vi "MeasurementServer_FourProbeMeasurement_WriteValue.vi"(0 "gRPCid":T3, 1 "FourProbeRawData":T1, 3 "error in (no error)":errorcluster) -> (10 "error out":errorcluster)   [LabVIEW 2019, in "labview-grpc-measurement-server.lvlib"]
uses:
  labview-grpc-measurement-server.lvlib
  MeasurementServer_gRPCid.ctl
  MeasurementServer_FourProbeRawData.ctl
  MeasurementServer_ErrorOutData.ctl
  <vilib>/Utility/error.llb/Error Cluster From Error Code.vi
  <vilib>/ErrorRing/Error Ring.xnode
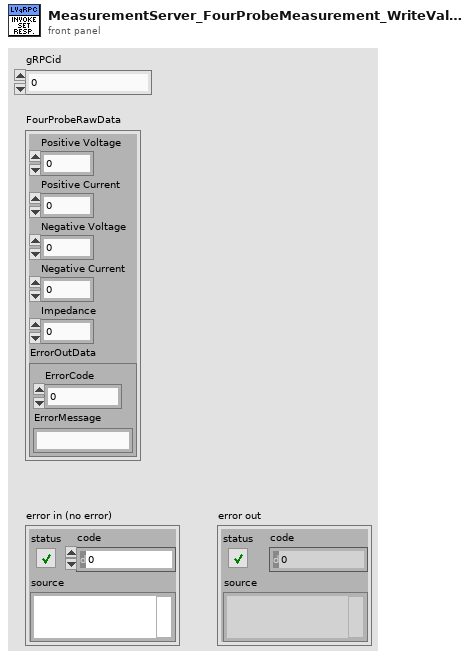
[diagram p1: front panel]
types:
  T1 = typedef "labview-grpc-measurement-server.lvlib/MeasurementServer_FourProbeRawData.ctl" = cluster{"Positive Voltage":dbl, "Positive Current":dbl, "Negative Voltage":dbl, "Negative Current":dbl, "Impedance":dbl, "ErrorOutData":T2}
  T2 = typedef "labview-grpc-measurement-server.lvlib/MeasurementServer_ErrorOutData.ctl" = cluster{"ErrorCode":i32, "ErrorMessage":string}
  T3 = typedef "labview-grpc-measurement-server.lvlib/MeasurementServer_gRPCid.ctl" = u64
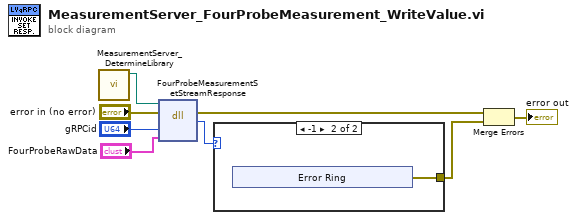
[diagram p0: block diagram]
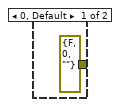
[diagram p2: hidden frame]
diagram:
  n1 = call "MeasurementServer_DetermineLibrary.vi"() -> ("path out"=w1:path)  [unwired: 11 in]
  n2 = dll-call lib="C:/dev/labview-grpc-measurement-server/build/Debug/labview_measurement_server.dll" fn="FourProbeMeasurementSetStreamResponse"(path in=w1, error in="error in (no error)", "id"="gRPCid", "data"="FourProbeRawData") -> (error out=w3:errorcluster, "return type"=w5:i32)  [unwired: 3 in, 1 out]
  n3 = case shown="-1" w5 {
    tunnel: [errorcluster {"status"=FALSE, "code"=0, "source"=""} ("error constant") w10] -> w4
    frame 0, Default {
    }
    frame -1 {
      n4 = xnode "Error Ring"() -> ("error out"=w10:errorcluster)
    }
  }
  n5 = Merge Errors(w3, w4) -> (→"error out":errorcluster)
